vi "FindAddresses.vi"(0 "Dali_usb_tridonics in":refnum<class "Dali_usb_tridonics.lvclass">, 3 "error in (no error)":errorcluster) -> (7 "Dali_usb_tridonics out":refnum<class "Dali_usb_tridonics.lvclass">, 8 "Devices_Addressed":i32, 10 "error out":errorcluster)   [LabVIEW 2014, in "Driver_interaction.lvlib" / "Dali_usb_tridonics.lvclass"]
uses:
  Dali_usb_tridonics.lvclass
  Controls/Commands enum.ctl
  Vendor/Controls/Addressing_type.ctl
  Dali_usb_tridonics.lvclass/Dali_usb_tridonics.ctl
  _Driver_interaction/_Driver_interaction.lvclass
  Vendor/Dali_usb.lvlib
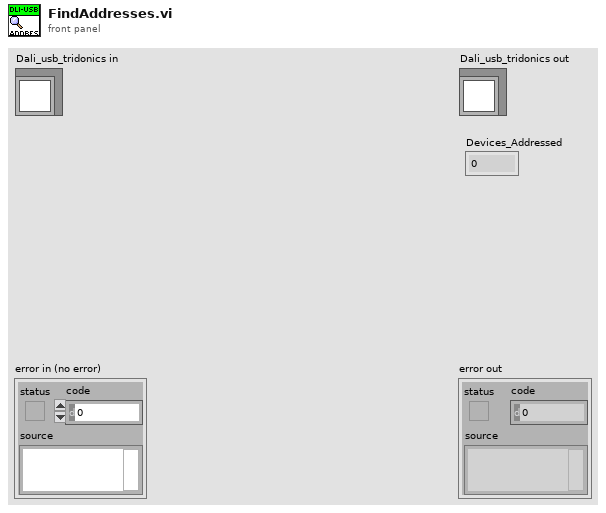
[diagram p1: front panel]
types:
  T1 = typedef "Dali_usb.lvlib/Addressing_type.ctl" = string
  T2 = typedef "Driver_interaction.lvlib/Dali_usb_tridonics.lvclass/Commands enum.ctl" = string
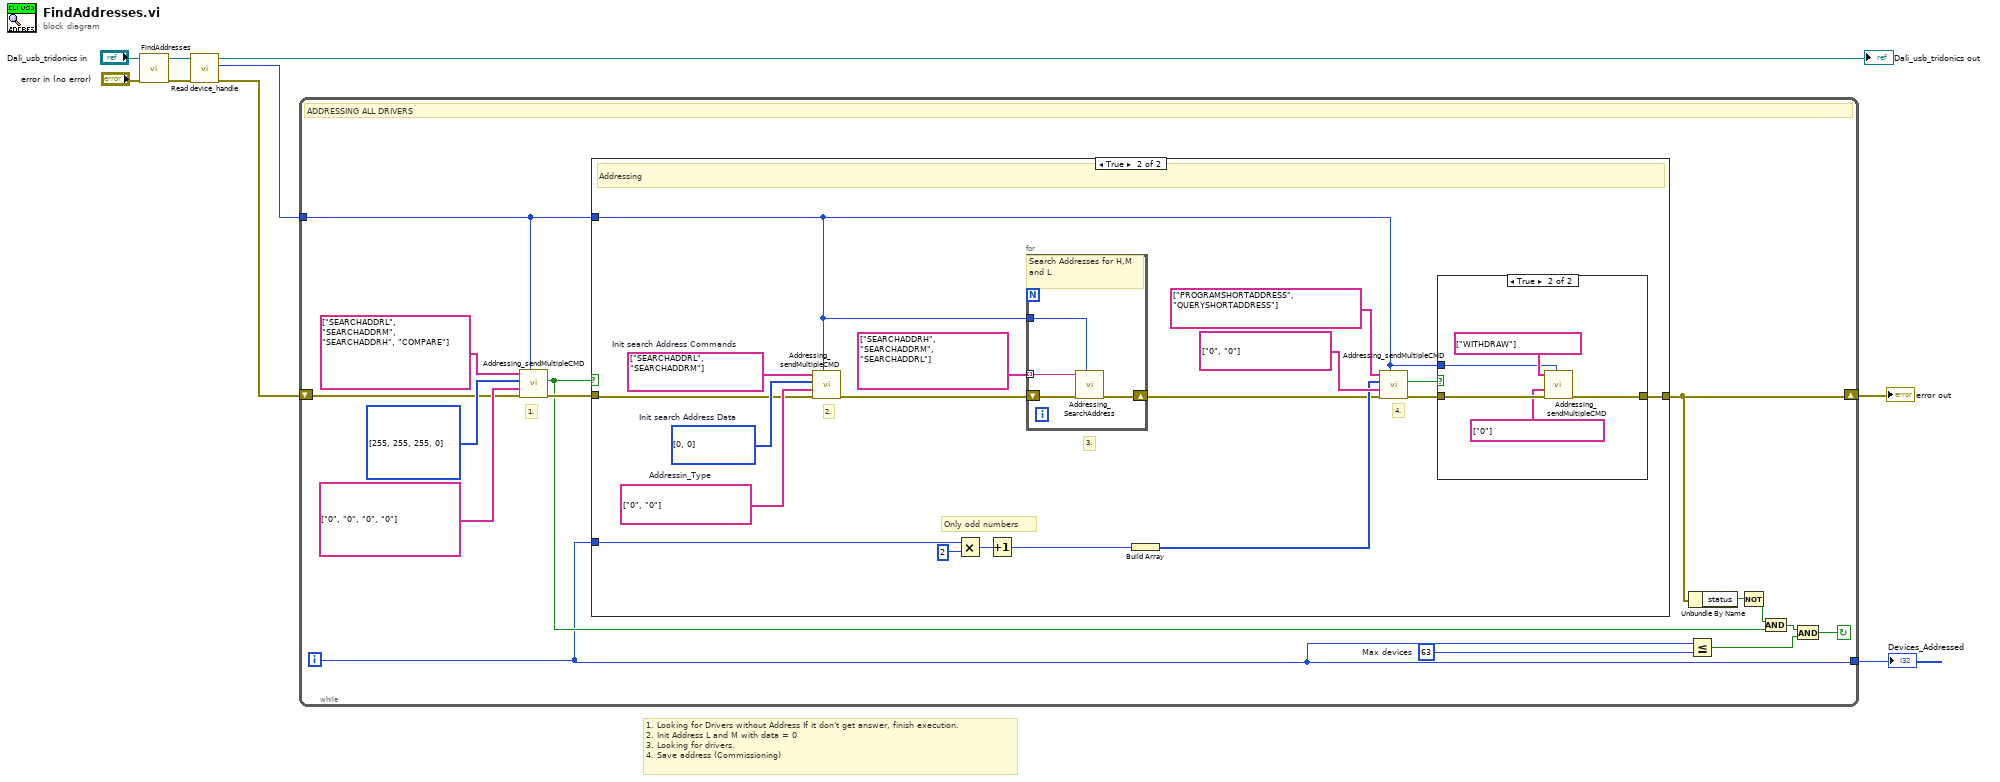
[diagram p0: block diagram]
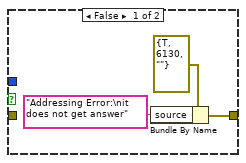
[diagram p3: hidden frame]
diagram:
  # "1. Looking for Drivers without Address If it don't get answer, finish execution.\n2. Init Address L and M with data = 0\n3. Looking for drivers.\n4. Save address (Commissioning)"
  n1 = call-parent "FindAddresses.vi"("_Driver_interaction in"="Dali_usb_tridonics in", "error in (no error)"="error in (no error)") -> ("_Driver_interaction out"=w6:refnum<class "Dali_usb_tridonics.lvclass">, "error out"=w4:errorcluster)  [unwired: 6 in, 1 out]
  n2 = call "Read device_handle.vi"("error in (no error)"=w4, "Dali_usb_tridonics in"=w6) -> ("error out"=w3:errorcluster, "device_handle"=w2:i32, "Dali_usb_tridonics out"=→"Dali_usb_tridonics out":refnum<class "Dali_usb_tridonics.lvclass">)  [unwired: 7 in]
  n3 = while {
    tunnel: w2 -> [w19]
    shift-right: [w18] -> w7
    shift-left: w3 -> [w21]
    tunnel: [w14] -> w1
    i -> [w14]
    stop <- w12 continue-if-true
    w13 = 63  # Max devices
    # "1."
    # "ADDRESSING ALL DRIVERS"
    n4 = call "Addressing_sendMultipleCMD.vi"("device_handle"=w19, "error in (no error)"=w21, "Addressin_Type"=T1[] ["0", "0", "0", "0"], "Data"=u32[] [255, 255, 255, 0] ("Check drivers Data"), "Commands"=T2[] ["SEARCHADDRL", "SEARCHADDRM", "SEARCHADDRH", "COMPARE"] ("Check drivers Commands")) -> ("error out"=w20:errorcluster, "Recieve Answer?"=w15:bool)  [unwired: 5 in]
    n5 = case shown="True" w15 {
      tunnel: w20 -> [w25 w39]
      tunnel: w19 -> [_ w26]
      tunnel: [w25 w28] -> w18
      tunnel: w14 -> [_ w32]
      frame False {
      }
      frame True {
        w40 = T1[] ["0", "0"]  # Addressin_Type
        w41 = u32[] [0, 0]  # Init search Address Data
        w42 = T2[] ["SEARCHADDRL", "SEARCHADDRM"]  # Init search Address Commands
        # "Only odd numbers"
        # "4."
        # "3."
        # "2."
        # "Addressing"
        n6 = call "Addressing_sendMultipleCMD.vi"("device_handle"=w26, "error in (no error)"=w39, "Addressin_Type"=w40, "Data"=w41, "Commands"=w42) -> ("error out"=w38:errorcluster)  [unwired: 5 in, 1 out]
        n7 = Multiply(x=w32, y=u32 2 ("x")) -> (x*y=w33:u32)
        n8 = Increment(x=w33) -> (x+1=w30:u32)
        n9 = for {
          tunnel: T2[] ["SEARCHADDRH", "SEARCHADDRM", "SEARCHADDRL"] -> [w55] mode=indexing
          tunnel: w26 -> [w53]
          shift-right: [w52] -> w34
          shift-left: w38 -> [w54]
          # "Search Addresses for H,M and L"
          n10 = call "Addressing_SearchAddress.vi"("device_handle"=w53, "error in (no error)"=w54, "Command"=w55) -> ("error out"=w52:errorcluster)  [unwired: 8 in]
        }
        n11 = Build Array(w30) -> (w35:u32[])
        n12 = call "Addressing_sendMultipleCMD.vi"("device_handle"=w26, "error in (no error)"=w34, "Addressin_Type"=T1[] ["0", "0"], "Data"=w35, "Commands"=T2[] ["PROGRAMSHORTADDRESS", "QUERYSHORTADDRESS"]) -> ("error out"=w29:errorcluster, "Recieve Answer?"=w27:bool)  [unwired: 5 in]
        n13 = case shown="True" w27 {
          tunnel: w29 -> [_ w51]
          tunnel: [w46 w50] -> w28
          tunnel: w26 -> [_ w47]
          frame False {
            n14 = Bundle By Name(cluster=errorcluster {"status"=TRUE, "code"=6130, "source"=""} ("error out"), "source"="Addressing Error:\nit does not get answer") -> (w46:errorcluster)
          }
          frame True {
            n15 = call "Addressing_sendMultipleCMD.vi"("device_handle"=w47, "error in (no error)"=w51, "Addressin_Type"=T1[] ["0"], "Commands"=T2[] ["WITHDRAW"]) -> ("error out"=w50:errorcluster)  [unwired: 6 in, 1 out]
          }
        }
      }
    }
    n16 = Unbundle By Name(w18) -> ("status"=w17:bool)
    n17 = Less Or Equal?(x=w14, y=w13) -> (x <= y?=w10:bool)
    n18 = Not(x=w17) -> (.not. x?=w16:bool)
    n19 = And(x=w16, y=w15) -> (x .and. y?=w11:bool)
    n20 = And(x=w11, y=w10) -> (x .and. y?=w12:bool)
  }
  "error out" <- w7
  "Devices_Addressed" <- w1
